vi "svm_delete_print_function.vi"(8 "error in (no error)":errorcluster) -> (0 "error out":errorcluster, 3 "User Event Out":refnum<user-event>)   [LabVIEW 2015]
uses:
  bin/x64/LabVIEW-libsvm.dll
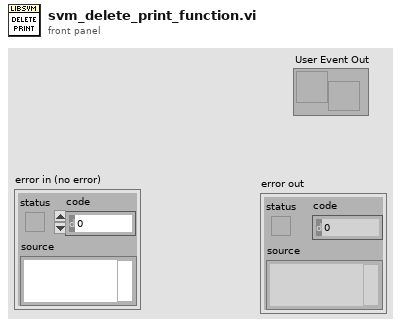
[diagram p1: front panel]
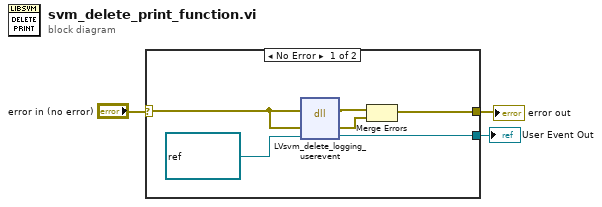
[diagram p0: block diagram]
diagram:
  n1 = case shown="No Error" "error in (no error)" {
    selector: "error in (no error)" -> [w9 w10]
    tunnel: [w6 w10] -> w3
    tunnel: [w4 _] -> w1
    frame No Error {
      n2 = dll-call lib="C:/dev/LabVIEW-libsvm/LabVIEW/bin/x64/LabVIEW-libsvm.dll" fn="LVsvm_delete_logging_userevent"(error in=w9, "lvErr"=w9, "loggingUserEvent_out"=refnum<user-event> refnum ("Logging event")) -> (error out=w8:errorcluster, "lvErr"=w7:errorcluster, "loggingUserEvent_out"=w4:refnum<user-event>)  [unwired: 3 in, 1 out]
      n3 = Merge Errors(w8, w7) -> (w6:errorcluster)
    }
    frame Error {
    }
  }
  "error out" <- w3
  "User Event Out" <- w1
